vi "Graph Cursor Update.vi"(5 "Waveform Ref in":T1, 7 "Timeline Ref in":T2, 8 "error in (no error)":errorcluster, 9 "Scale graph X-axis (T)":bool=TRUE, 11 "Xinformation In":T3) -> (0 "error out":errorcluster, 2 "Waveform Ref out":T1, 3 "Xinformation Out":T3)   [LabVIEW 2017, in "XGrapher.xctl"]
doc: "Redraws the main waveform graph by using the cursor positions to update the waveform's scale range."
uses:
  XGrapher.xctl
  Typedefs/Xinformation.ctl
  Typedefs/Xcrtl-Click Operation.ctl
  Typedefs/Xctrl-Timeline graph ref.ctl
  Typedefs/Xctrl-Waveform graph ref.ctl
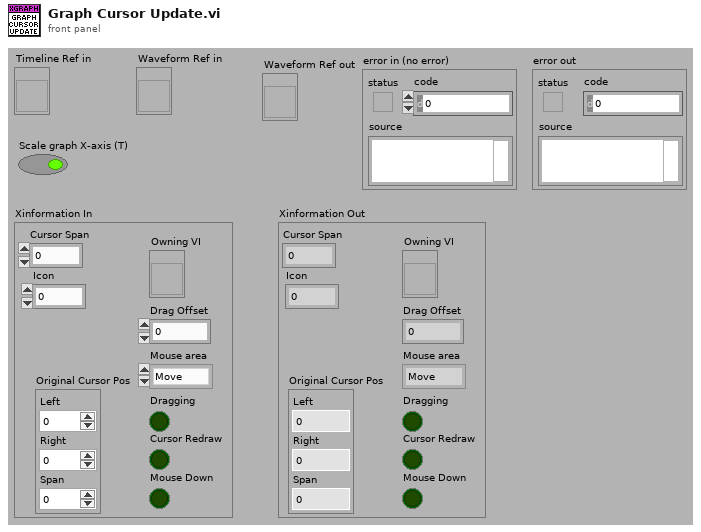
[diagram p1: front panel]
types:
  T1 = typedef "XGrapher.xctl/Xctrl-Waveform graph ref.ctl" = refnum<vi>
  T2 = typedef "XGrapher.xctl/Xctrl-Timeline graph ref.ctl" = refnum<vi>
  T3 = typedef "XGrapher.xctl/Xinformation.ctl" = cluster{"Cursor Span":dbl, "Icon":u16, "Mouse Down":bool, "Owning VI":refnum<vi>, "Mouse area":T4, "Dragging":bool, "Drag Offset":dbl, "Original Cursor Pos":cluster{"Left":dbl, "Right":dbl, "Span":dbl}, "Cursor Redraw":bool}
  T4 = typedef "XGrapher.xctl/Xcrtl-Click Operation.ctl" = enum16{"Move", "left cursor", "right cursor", "none"}
  T5 = typedef "LVRangeTypeDef.ctl" = cluster{"Minimum":dbl, "Maximum":dbl, "Increment":dbl, "Minor Increment":dbl, "Start":dbl}
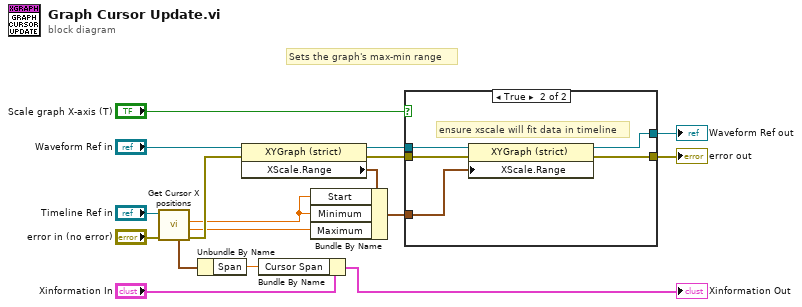
[diagram p0: block diagram]
diagram:
  # "Sets the graph's max-min range"
  n1 = call "Get Cursor X positions.vi"("error in"="error in (no error)", "Timeline Graph"="Timeline Ref in") -> ("error out"=w13:errorcluster, "Right cursor pos."=w7:dbl, "Left cursor pos."=w6:dbl, "Cursors"=w8:cluster{"Left":dbl, "Right":dbl, "Span":dbl})  [unwired: 5 in, 1 out]
  n2 = Unbundle By Name(w8) -> ("Span"=w11:dbl)
  n3 = property on="Property Node" class="XYGraph (strict)"(reference="Waveform Ref in", error in=w13) -> (reference out=w4:T1, error out=w2:errorcluster, "XScale.Range"=w1:T5)
  n4 = Bundle By Name(cluster="Xinformation In", "Cursor Span"=w11) -> (→"Xinformation Out":T3)
  n5 = Bundle By Name(cluster=w1, "Start"=w6, "Minimum"=w6, "Maximum"=w7) -> (w3:T5)
  n6 = case shown="True" "Scale graph X-axis (T)" {
    tunnel: [w19 w24] -> w12
    tunnel: w4 -> [w18 w23]
    tunnel: w3 -> [_ w22]
    tunnel: w2 -> [w19 w21]
    tunnel: [w18 w20] -> w5
    frame False {
    }
    frame True {
      # "ensure xscale will fit data in timeline"
      n7 = property on="Property Node" class="XYGraph (strict)"(reference=w23, error in=w21, "XScale.Range"=w22) -> (reference out=w20:T1, error out=w24:errorcluster)
    }
  }
  "error out" <- w12
  "Waveform Ref out" <- w5
